vi "Test Copy Array To Image ARGB.vi"(8 "error in (no error)":errorcluster, 11 "Test Case In":refnum<class "01_Image.lvclass">) -> (0 "error out":errorcluster, 3 "Test Case Out":refnum<class "01_Image.lvclass">)   [LabVIEW 2020, in "test.lvlib" / "01_Image.lvclass"]
uses:
  01_Image.lvclass
  C:/Program Files (x86)/National Instruments/LabVIEW 2020/vi.lib/Astemes/LUnit/Test Case.lvclass
  common/Image Size (Integer).ctl
  <vilib>/Astemes/LUnit/Test Case.lvclass/Test Case.ctl
  image/New Image (ARGB Preallocated).vi
  4993e8ee-a06a-463a-9684-69129f64d5ce.vi
  image/Copy Array to Image.vi
  image/New Image (ARGB Preallocated).vi/3321fa97-f432-4e1e-8db9-a0df79aed21b.vi
  image/ARGB Colour to U32 Pixel Value.vi
  <vilib>/Astemes/LUnit/Core/LUnit Test Case/Private/Append Pass Result.vi
  <vilib>/Astemes/LUnit/Core/LUnit Test Case/Private/Append Fail Result.vi
  4993e8ee-a06a-463a-9684-69129f64d5ce.vi/9c5d11cd-9439-4240-a1ee-d9baace9c924.vi
  <vilib>/Astemes/LUnit/Core/LUnit Test Case/Private/Run In UI.vi
  <vilib>/Utility/error.llb/Clear Errors.vi
  <vilib>/Utility/error.llb/Error Cluster From Error Code.vi
  <vilib>/picture/pixmap.llb/Flatten Pixmap.vi
  image/image.lvlib
  common/common.lvlib
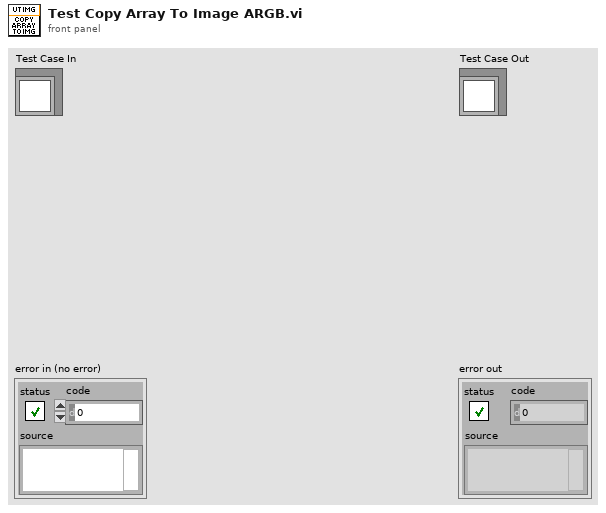
[diagram p1: front panel]
types:
  T1 = typedef "common.lvlib/Image Size (Integer).ctl" = cluster{"Width":u16, "Height":u16}
  T2 = typedef "image.lvlib/ARGB Image.ctl" = refnum<data-value>
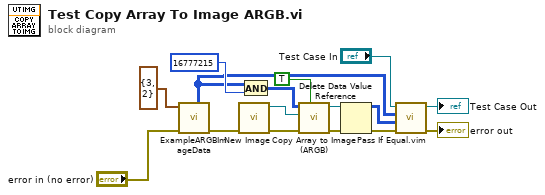
[diagram p0: block diagram]
diagram:
  n1 = call "ExampleARGBImageData.vi"("error in (no error)"="error in (no error)", "Image Size"=T1 {"Width"=3, "Height"=2}) -> ("error out"=w6:errorcluster, "ARGB Array Data"=w2:u32[][])  [unwired: 6 in, 2 out]
  n2 = call-poly "New Image.vi"("error in (no error)"=w6) -> ("error out"=w11:errorcluster, "ARGB Image"=w10:T2)  [unwired: 9 in]
  n3 = And(x=w2, y=u32 16777215) -> (x .and. y?=w4:u32[][])
  n4 = call "Copy Array to Image (ARGB).vi"("Set Alpha Values to 255 (Default: True)"=TRUE, "error in (no error)"=w11, "ARGB Image Destination in"=w10, "U32 ARBG Data"=w4) -> ("error out"=w9:errorcluster, "ARGB Image Destination"=w8:T2)  [unwired: 6 in]
  n5 = Delete Data Value Reference(data value reference=w8, error in=w9) -> (data value=w13:u32[][], error out=w12:errorcluster)
  n6 = call "Pass If Equal.vim"("error in (no error)"=w12, "Actual"=w13, "Expected"=w2, "LUnit Test Case In"="Test Case In") -> ("error out"=→"error out":errorcluster, "LUnit Test Case Out"=→"Test Case Out":refnum<class "01_Image.lvclass">)  [unwired: 6 in]
